vi "APU + Knock.vi"() -> ()   [LabVIEW 2013]
uses:
  IP Source/APU/Settings.ctl
  IP Source/APU/Input.ctl
  IP Source/APU/Output.ctl
  IP Source/Knock Sensor/Generate Settings.ctl
  IP Source/Knock Sensor/Cylinder Settings.ctl
  IP Source/APU/Shared Settings.ctl
  IP Source/Knock Sensor/Cylinder Input.ctl
  IP Source/Knock Sensor/Generate Input.ctl
  <vilib>/Platform/TimedLoop/XDataNode/timing_clust.ctl
  <vilib>/Platform/TimedLoop/XDataNode/nitl_modes.ctl
  <vilib>/Platform/TimedLoop/XDataNode/wakeup.ctl
  <vilib>/rvi/Emulation/niFpgaSctlEmulationGetInTimedLoop.vi
  <vilib>/rvi/Emulation/niFpgaEmulationReportErrorSimple.vi
  <vilib>/rvi/Emulation/niFpgaGetClockAttributes.vi
  <vilib>/rvi/DataTransferAndStorage/Container/Common/niFpgaContainerExecOnDevCompGetState.vi
  <vilib>/rvi/DataTransferAndStorage/Register/Emulation/niFpgaRegisterEmulationFpgaImpl.vi
  <instcachedir>/0/niFpgaRegisterEmulationFpgaImpl_DCF4BC0110594B98B44A971D60CEEC4D.lvgen/niFpgaRegisterEmulationFpgaImpl_DCF4BC0110594B98B44A971D60CEEC4D_006.vi
  <vilib>/rvi/DataTransferAndStorage/Container/Common/niFpgaContainerGetUniqueNameForEmu.vi
  <vilib>/rvi/interface/RandomDataEmulation/nirviRandomDataFPGAFIFO.vi
  <vilib>/rvi/interface/RandomDataEmulation/niFpgaRandomDataHandleErrors.vi
  <vilib>/rvi/Emulation/niFpgaCriticalErrorInLSC.vi
  <vilib>/Platform/TimedLoop/XDataNode/XDataNode.xnode
  <vilib>/rvi/DataTransferAndStorage/Container/XNode/niFpgaContainer.xnode
  <vilib>/rvi/DataTransferAndStorage/Register/Emulation/niFpgaRegisterEmulationRefIn.vi
  <vilib>/rvi/interface/RandomDataEmulation/nirviRandomDataFpgaReadWriteTemplate.vi
  <vilib>/Platform/TimedLoop/XDataNode/XDNodeRunTimeDep.lvlib
  IP Source/APU/APU.lvlib
  IP Source/Knock Sensor/Knock Sensor.lvlib
panel:
  in  "input.Knock AO0":T1
  in  "input.Knock AO0.Cylinder 4":T2
  in  "input.Knock AO0.Cylinder 3":T2
  in  "input.Knock AO0.Cylinder 2":T2
  in  "input.Knock AO0.Cylinder 1":T2
  in  "shared settings.my apu":T3 {"cycle start" format="%#.15g"}
  out "Knock Signal":i16
  out "Timed Out?":bool
  in  "settings.Knock AO0.Cylinder 4":T4
  in  "settings.Knock AO0.Cylinder 3":T4
  in  "settings.Knock AO0.Cylinder 2":T4
  in  "settings.Knock AO0.Cylinder 1":T4
  in  "settings.Knock AO0":T5
  out "Output.my apu":T6 caption="output"
  in  "Input.my apu":T7={"desired speed"=0.0, "reset"=TRUE} caption="input"
  in  "Settings.my apu":T8 caption="settings"
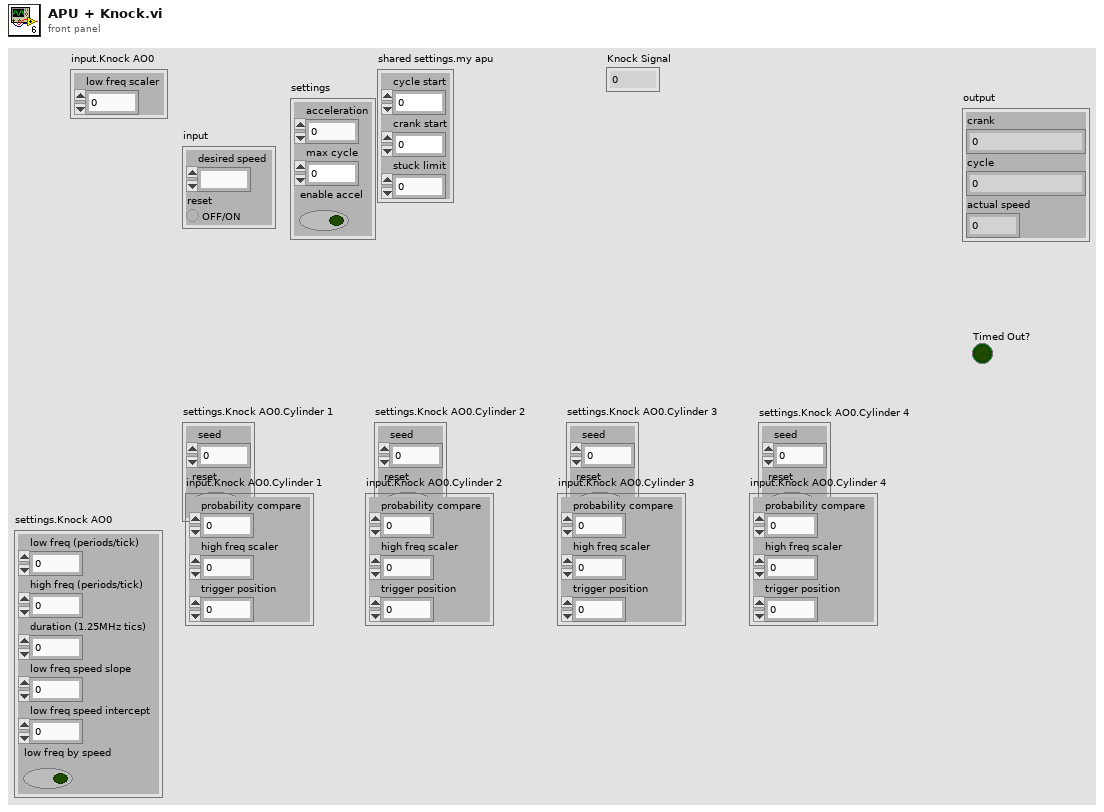
[diagram p1: front panel]
types:
  T1 = typedef "Engine Simulation Toolkit.lvlib/Knock Sensor.lvlib/Generate Input.ctl" = cluster{"low freq scaler":fxp<+,10,0>}
  T2 = typedef "Engine Simulation Toolkit.lvlib/Knock Sensor.lvlib/Cylinder Input.ctl" = cluster{"probability compare":u16, "high freq scaler":fxp<+,10,0>, "trigger position":u16}
  T3 = typedef "Engine Simulation Toolkit.lvlib/APU.lvlib/Shared Settings.ctl" = cluster{"cycle start":fxp<+,2,2>, "crank start":u16, "stuck limit":fxp<+,18,18>}
  T4 = typedef "Engine Simulation Toolkit.lvlib/Knock Sensor.lvlib/Cylinder Settings.ctl" = cluster{"seed":u16, "reset":bool}
  T5 = typedef "Engine Simulation Toolkit.lvlib/Knock Sensor.lvlib/Generate Settings.ctl" = cluster{"low freq (periods/tick)":fxp<+,32,0>, "high freq (periods/tick)":fxp<+,32,0>, "duration (1.25MHz tics)":fxp<+,18,18>, "low freq speed slope":fxp<+,16,-3>, "low freq speed intercept":fxp<+,10,-10>, "low freq by speed":bool}
  T6 = typedef "Engine Simulation Toolkit.lvlib/APU.lvlib/Output.ctl" = cluster{"crank":u16, "cycle":u16, "actual speed":fxp<+/-,23,2>}
  T7 = typedef "Engine Simulation Toolkit.lvlib/APU.lvlib/Input.ctl" = cluster{"desired speed":fxp<+/-,23,2>, "reset":bool}
  T8 = typedef "Engine Simulation Toolkit.lvlib/APU.lvlib/Settings.ctl" = cluster{"acceleration":fxp<+,18,-20>, "max cycle":fxp<+,2,2>, "enable accel":bool}
  T9 = typedef "Engine Simulation Toolkit.lvlib/APU.lvlib/Register Bus.ctl" = cluster{"Speed":refnum<k21>, "Crank Angle":refnum<k21>, "Cycle Angle":refnum<k21>, "Crank Count":refnum<k21>, "Cycle Count":refnum<k21>, "1.25 MHz Counter":refnum<k21>, "shared settings":T3}
  T10 = typedef "XDNodeRunTimeDep.lvlib/timing_clust.ctl" = cluster{"Expected End [f-1]":u64, "Actual End [f-1]":u64, "Finished Late? [f-1]":bool, "Expected End [i-1]":u64, "Actual End [i-1]":u64, "Finished Late? [i-1]":bool, "Expected Start [i]":u64, "Actual Start [i]":u64, "Expected Start [f]":u64, "Actual Start [f]":u64, "Source Name":string, "Structure Name":string, "Period":i64, "Deadline":i64, "Offset":i64, "Start":i64, "Priority":i32, "Timeout":i32, "Mode":T11, "Wakeup Reason":T12, "Error":errorcluster, "Source Type":string, "Secondary Source Type":string, "Global End Time":u64, "Global Start Time":u64, "Frame Duration":u64, "Iteration Duration":u64, "Assigned CPU":i32, "I/O Scan Engine Mode":u32}
  T11 = typedef "XDNodeRunTimeDep.lvlib/nitl_modes.ctl" = enum32{"No Change", "Process missed periods, maintain original phase", "Discard missed periods, maintain original phase", "Process missed periods, ignore original phase", "Discard missed periods, ignore original phase"}
  T12 = typedef "XDNodeRunTimeDep.lvlib/wakeup.ctl" = enum32{"Normal", "Aborted", "Asynchronous wakeup", "Timing source error", "Timed loop error", "Timeout"}
  T13 = typedef "Engine Simulation Toolkit.lvlib/Knock Sensor.lvlib/Triggered Cylinder Data.ctl" = cluster{"trigger knock":bool, "high freq scaler":fxp<+,10,0>}
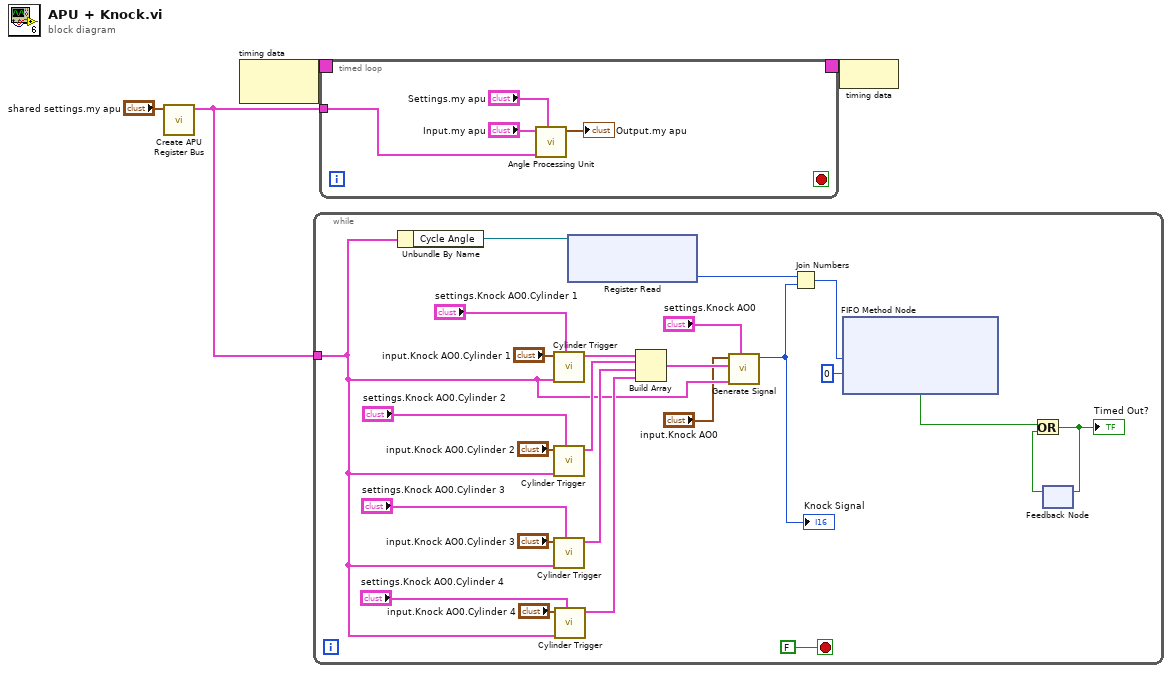
[diagram p0: block diagram]
diagram:
  n1 = call "Create APU Register Bus.vi"("shared settings.<user name>"="shared settings.my apu") -> ("register bus"=w2:T9)  [unwired: 10 in]
  n2 = node-c288() -> (w4:T10)  [unwired: 1 in]
  n3 = while {
    tunnel: w2 -> [w7]
    stop <- FALSE stop-if-true
    n4 = Unbundle By Name(w7) -> ("Cycle Angle"=w19:refnum<k21>)
    n5 = call "Cylinder Trigger.vi"("settings.<user name>"="settings.Knock AO0.Cylinder 1", "register bus"=w7, "input.<user name>"="input.Knock AO0.Cylinder 1") -> ("triggered knock data"=w29:T13)  [unwired: 8 in]
    n6 = call "Cylinder Trigger.vi"("settings.<user name>"="settings.Knock AO0.Cylinder 2", "register bus"=w7, "input.<user name>"="input.Knock AO0.Cylinder 2") -> ("triggered knock data"=w28:T13)  [unwired: 8 in]
    n7 = call "Cylinder Trigger.vi"("settings.<user name>"="settings.Knock AO0.Cylinder 3", "register bus"=w7, "input.<user name>"="input.Knock AO0.Cylinder 3") -> ("triggered knock data"=w27:T13)  [unwired: 8 in]
    n8 = call "Cylinder Trigger.vi"("settings.<user name>"="settings.Knock AO0.Cylinder 4", "register bus"=w7, "input.<user name>"="input.Knock AO0.Cylinder 4") -> ("triggered knock data"=w26:T13)  [unwired: 8 in]
    n9 = xnode ("Register Read")("Register In"=w19) -> ("Data"=w18:u16)  [unwired: 1 out]
    n10 = Build Array(w29, w28, w27, w26) -> (w25:T13[])
    n11 = call "Generate Signal.vi"("settings.<user name>"="settings.Knock AO0", "register bus"=w7, "triggered knock data"=w25, "input.<user name>"="input.Knock AO0") -> ("knock signal"=w17:i16)  [unwired: 7 in]
    "Knock Signal" <- w17
    n12 = Join Numbers(hi=w18, lo=w17) -> ((hi.lo)=w16:u32)
    n13 = xnode ("FIFO Method Node")("Element"=w16, "Timeout"=0) -> ("Timed Out?"=w22:bool)  [unwired: 1 in, 1 out]
    n14 = feedback #1() -> (w21:bool)  [unwired: 1 in]
    n15 = Or(x=w22, y=w21) -> (x .or. y?=w20:bool)
    "Timed Out?" <- w20
    n16 = feedback-in #1(w20) -> ()
  }
  n17 = timed-loop {
    timing: w4 -> [_]
    timing-out: [_] -> w3
    tunnel: w2 -> [w30]
    stop <- _ stop-if-true
    n18 = call "Angle Processing Unit.vi"("settings.<user name>"="Settings.my apu", "register bus"=w30, "input.<user name>"="Input.my apu") -> ("output.<user name>"=→"Output.my apu":T6)  [unwired: 8 in]
  }
  n19 = node-c288(w3) -> ()
